vi "sub-set menu short key.vi"(8 "error in (no error)":errorcluster caption="错误输入（无错误）", 11 "menubar in":refnum<k9>) -> (0 "error out":errorcluster caption="错误输出", 3 "menubar out":refnum<k9>)   [LabVIEW 2011]
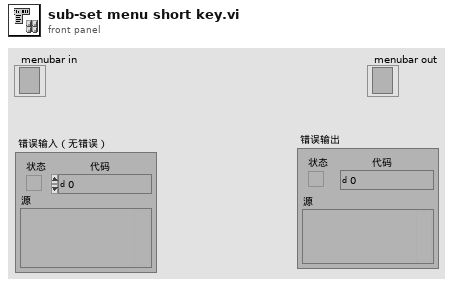
[diagram p1: front panel]
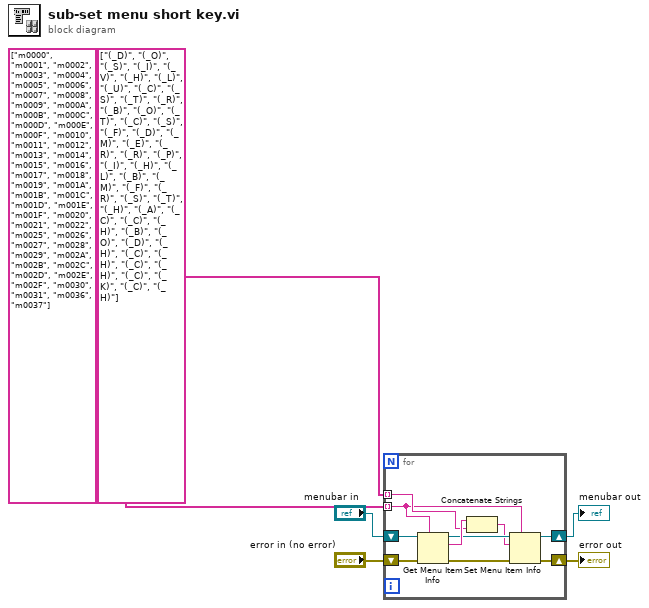
[diagram p0: block diagram]
diagram:
  n1 = for {
    tunnel: string[] ["m0000", "m0001", "m0002", "m0003", "m0004", "m0005", "m0006", "m0007", "m0008", "m0009", "m000A", "m000B", "m000C", "m000D", "m000E", "m000F", "m0010", "m0011", "m0012", "m0013", "m0014", "m0015", "m0016", "m0017", "m0018", "m0019", "m001A", "m001B", "m001C", "m001D", "m001E", "m001F", "m0020", "m0021", "m0022", "m0025", "m0026", "m0027", "m0028", "m0029", "m002A", "m002B", "m002C", "m002D", "m002E", "m002F", "m0030", "m0031", "m0036", "m0037"] -> [w11] mode=indexing
    tunnel: string[] ["(_D)", "(_O)", "(_S)", "(_I)", "(_V)", "(_H)", "(_L)", "(_U)", "(_C)", "(_S)", "(_T)", "(_R)", "(_B)", "(_O)", "(_T)", "(_C)", "(_S)", "(_F)", "(_D)", "(_M)", "(_E)", "(_R)", "(_R)", "(_P)", "(_I)", "(_H)", "(_L)", "(_B)", "(_M)", "(_F)", "(_R)", "(_S)", "(_T)", "(_H)", "(_A)", "(_C)", "(_C)", "(_H)", "(_B)", "(_O)", "(_D)", "(_H)", "(_C)", "(_H)", "(_C)", "(_H)", "(_C)", "(_K)", "(_C)", "(_H)"] -> [w14] mode=indexing
    shift-right: [w10] -> w3
    shift-left: "menubar in" -> [w16]
    shift-right: [w7] -> w1
    shift-left: "error in (no error)" -> [w9]
    n2 = Get Menu Item Info(7:w11, 8:w9, 11:w16) -> (0:w8:errorcluster, 2:w15:string, 3:w13:refnum<k9>)  [unwired: 4 out]
    n3 = Concatenate Strings(w15, w14) -> (w12:string)
    n4 = Set Menu Item Info(7:w11, 8:w8, 10:w12, 11:w13) -> (0:w7:errorcluster, 3:w10:refnum<k9>)  [unwired: 3 in]
  }
  "menubar out" <- w3
  "error out" <- w1
